vi "p, q, t, a e b.vi"(1 "Infos para processamento":T1={"Diâmetro do furo [mm]"=1.4, "Diâmetro da linha média [mm]"=5.0, "IncF"=0.2, "Módulo de elasticidade [GPa]"=207.0, "Módulo de Poisson"=0.3, "Tipo de roseta utilizada"=enum."Tipo A", "Método de análise"=enum."Simplificado 2008", "Pfinal"=0.3, "Parar auto."=TRUE}, 2 "Dados in":T3) -> (0 "Dados out":T2)   [LabVIEW 2016]
uses:
  Controles/p,q, t, a e b.ctl
  Controles/Infos para processamento.ctl
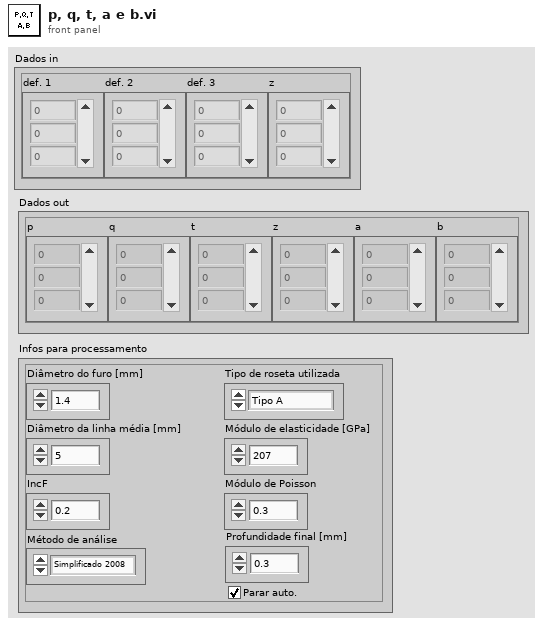
[diagram p1: front panel]
types:
  T1 = typedef "Infos para processamento.ctl" = cluster{"Diâmetro do furo [mm]":dbl, "Diâmetro da linha média [mm]":dbl, "IncF":dbl, "Módulo de elasticidade [GPa]":dbl, "Módulo de Poisson":dbl, "Tipo de roseta utilizada":enum16{"Tipo A", "Tipo B", "Tipo C"}, "Método de análise":enum16{"Não uniforme 2013", "Simplificado 2013", "Simplificado 2008"}, "Pfinal":dbl, "Parar auto.":bool}
  T2 = typedef "p,q, t, a e b.ctl" = cluster{"p":dbl[], "q":dbl[], "t":dbl[], "z":dbl[], "a":dbl[], "b":dbl[]}
  T3 = typedef "Deformações.ctl" = cluster{"def. 1 ":dbl[], "def. 2":dbl[], "def. 3":dbl[], "z":dbl[]}
  T4 = enum16{"Não uniforme 2013", "Simplificado 2013", "Simplificado 2008"}
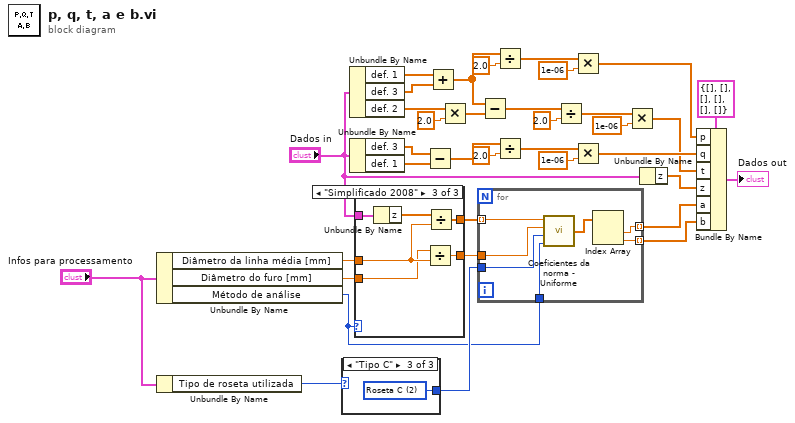
[diagram p0: block diagram]
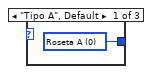
[diagram p2: hidden frame]
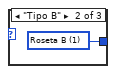
[diagram p3: hidden frame]
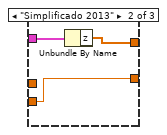
[diagram p5: hidden frame]
diagram:
  n1 = Unbundle By Name("Infos para processamento") -> ("Diâmetro da linha média [mm]"=w6:dbl, "Diâmetro do furo [mm]"=w5:dbl, "Método de análise"=w1:T4)
  n2 = Unbundle By Name("Infos para processamento") -> ("Tipo de roseta utilizada"=w3:enum16{"Tipo A", "Tipo B", "Tipo C"})
  n3 = case shown="\"Tipo C\"" w3 {
    tunnel: [w37 w38 w39] -> w2
    frame "Tipo A", Default {
      w37 = u16 0 items=["Roseta A", "Roseta B", "Roseta C"] ("Tipo de roseta")
    }
    frame "Tipo B" {
      w38 = u16 1 items=["Roseta A", "Roseta B", "Roseta C"] ("Tipo de roseta")
    }
    frame "Tipo C" {
      w39 = u16 2 items=["Roseta A", "Roseta B", "Roseta C"] ("Tipo de roseta")
    }
  }
  n4 = Unbundle By Name("Dados in") -> ("def. 1"=w19:dbl[], "def. 3"=w20:dbl[], "def. 2"=w12:dbl[])
  n5 = Unbundle By Name("Dados in") -> ("def. 3"=w22:dbl[], "def. 1"=w23:dbl[])
  n6 = case shown="\"Simplificado 2008\"" w1 {
    tunnel: [_ w41 w48] -> w11
    tunnel: w6 -> [_ _ w47]
    tunnel: [_ w40 w46] -> w10
    tunnel: w5 -> [_ w40 w45]
    tunnel: "Dados in" -> [_ w42 w43]
    frame "Não uniforme 2013", Default {
    }
    frame "Simplificado 2013" {
      n7 = Unbundle By Name(w42) -> ("z"=w41:dbl[])
    }
    frame "Simplificado 2008" {
      n8 = Unbundle By Name(w43) -> ("z"=w44:dbl[])
      n9 = Divide(x=w45, y=w47) -> (x/y=w46:dbl)
      n10 = Divide(x=w44, y=w47) -> (x/y=w48:dbl[])
    }
  }
  n11 = Subtract(x=w22, y=w23) -> (x-y=w24:dbl[])
  n12 = Add(x=w19, y=w20) -> (x+y=w25:dbl[])
  n13 = Multiply(x=w12, y=2.0) -> (x*y=w27:dbl[])
  n14 = for {
    tunnel: w11 -> [w54] mode=indexing
    tunnel: w10 -> [w53]
    tunnel: w2 -> [w52]
    tunnel: [w55] -> w8 mode=indexing
    tunnel: [w50] -> w7 mode=indexing
    tunnel: w1 -> [w49]
    n15 = call "Coeficientes da norma - Uniforme.vi"("Método de análise"=w49, "Tipo de roseta"=w52, "Coluna"=w53, "Linha"=w54) -> ("Coeficiente a e b"=w51:dbl[])
    n16 = Index Array(array=w51) -> (element #1=w55:dbl, element #2=w50:dbl)  [unwired: 2 in]
  }
  n17 = Subtract(x=w25, y=w27) -> (x-y=w28:dbl[])
  n18 = Divide(x=w25, y=2.0) -> (x/y=w32:dbl[])
  n19 = Divide(x=w24, y=2.0) -> (x/y=w36:dbl[])
  n20 = Divide(x=w28, y=2.0) -> (x/y=w34:dbl[])
  n21 = Multiply(x=w32, y=1e-06 ("Diâmetro da roseta")) -> (x*y=w17:dbl[])
  n22 = Multiply(x=w36, y=1e-06 ("Diâmetro da roseta")) -> (x*y=w16:dbl[])
  n23 = Multiply(x=w34, y=1e-06 ("Diâmetro da roseta")) -> (x*y=w15:dbl[])
  n24 = Unbundle By Name("Dados in") -> ("z"=w14:dbl[])
  n25 = Bundle By Name(cluster=T2 {"p"=[], "q"=[], "t"=[], "z"=[], "a"=[], "b"=[]} ("Dados"), "p"=w17, "q"=w16, "t"=w15, "z"=w14, "a"=w8, "b"=w7) -> (→"Dados out":T2)
